vi "Combination_Digitizer_Driver - REWORK.vi"(0 "Mode":T5(ring), 1 "Horizontal Settings":T2={"number of records"=1, "reference position"=50.0, "min record length"=50000, "min sample rate"=200000.0, "enforce realtime"=FALSE, "maximum input frequency"=0.0} {"maximum input frequency" format="%.2f"; "min sample rate" step=1000000.0; "reference position" format="%.1f"; "number of records" step=1}, 2 "Vertical Settings":T4={"vertical coupling"=enum."DC", "probe attenuation"=20.0, "vertical range"=120.0, "vertical offset"=0.0} {"vertical offset" format="%.4f"; "vertical range" format="%.2f"; "probe attenuation" format="%.1f"}, 3 "Trigger Settings":T3={"trigger level"=30.0, "trigger type"=enum."Edge", "Trigger Source"=enum."Channel 0", "Trigger Slope"=enum."Positive"} {"trigger level" format="%.2f"}, 5 "Channel Name":string="0", 11 "error in":errorcluster) -> (6 "Waveform Array":waveform(dbl)[](array[waveform]), 8 "Ch1_Plot":dbl[](array[numeric]), 15 "error out":errorcluster)   [LabVIEW 2010]
uses:
  Typedef-Channel Parameters.ctl
panel:
  in  "Channel Parameters In":T1={"Channel Name"="0", "Number of Records"=0, "Reference Position"=0.0, "Minimum Record Length"=0, "Minimum Sample Rate"=0.0, "Maximum Input Frequency"=0.0, "Enforce Realtime"=FALSE, "Vertical Coupling"=enum."AC", "Probe Attenuation"=0.0, "Vertical Range (V)"=0.0, "Vertical Offset"=0.0, "Trigger Level"=0.0, "Trigger Type"=enum."Edge", "Trigger Source"=enum."Immediate", "Trigger Slope"=enum."Positive", "Digitizer 1 Used?"=FALSE, "Digitizer 1 Channels"="", "Digitizer 1 Reference"="", "Digitizer 1 Gain Multiplier"=nan, "Digitizer 2 Used?"=FALSE, "Digitizer 2 Channels"="", "Digitizer 2 Reference"="", "Session References"=[]}
  out "Channel Parameters":T1={"Channel Name"="0", "Number of Records"=0, "Reference Position"=0.0, "Minimum Record Length"=0, "Minimum Sample Rate"=0.0, "Maximum Input Frequency"=0.0, "Enforce Realtime"=FALSE, "Vertical Coupling"=enum."AC", "Probe Attenuation"=0.0, "Vertical Range (V)"=0.0, "Vertical Offset"=0.0, "Trigger Level"=0.0, "Trigger Type"=enum."Edge", "Trigger Source"=enum."Immediate", "Trigger Slope"=enum."Positive", "Digitizer 1 Used?"=FALSE, "Digitizer 1 Channels"="", "Digitizer 1 Reference"="", "Digitizer 1 Gain Multiplier"=nan, "Digitizer 2 Used?"=FALSE, "Digitizer 2 Channels"="", "Digitizer 2 Reference"="", "Session References"=[]}
  out "Waveform":T6(graph)
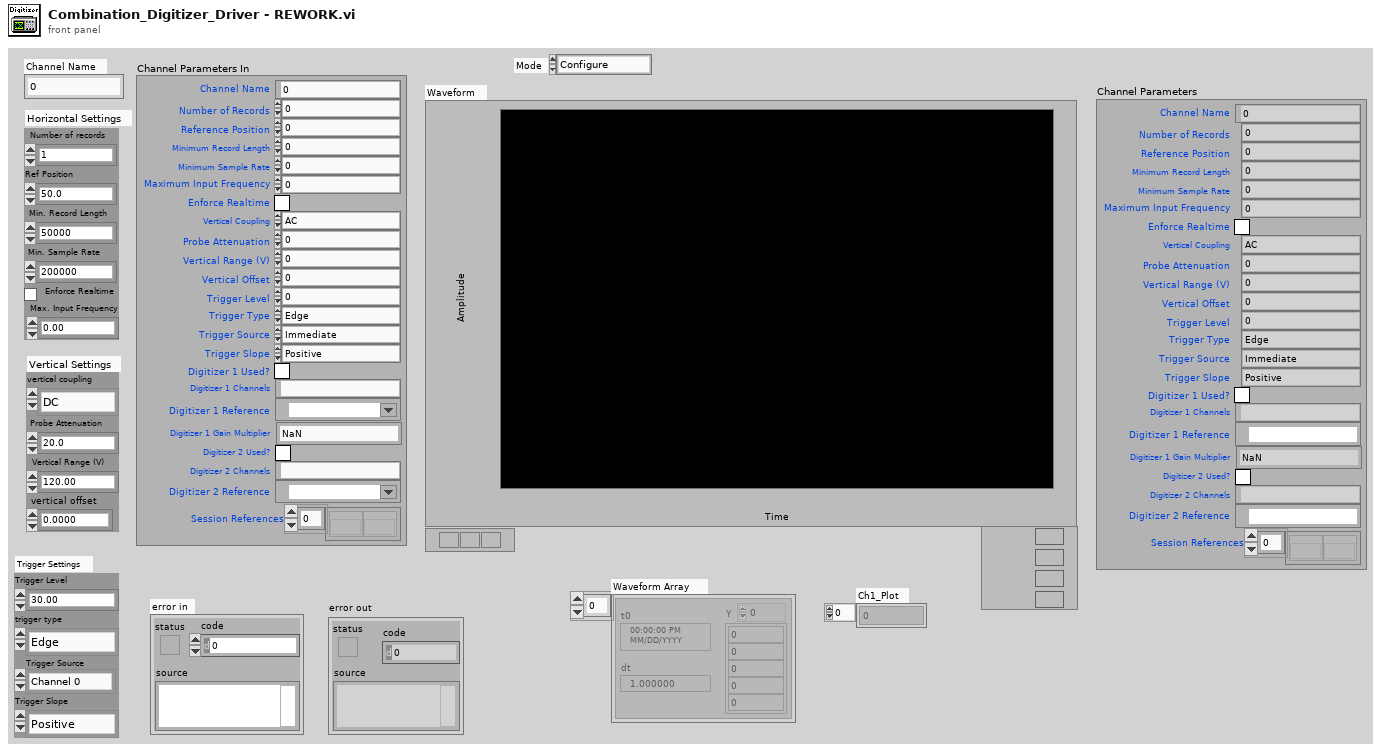
[diagram p1: front panel]
types:
  T1 = typedef "Typedef-Channel Parameters.ctl" = cluster{"Channel Name":string, "Number of Records":i32, "Reference Position":dbl, "Minimum Record Length":i32, "Minimum Sample Rate":dbl, "Maximum Input Frequency":dbl, "Enforce Realtime":bool, "Vertical Coupling":enum16{"AC", "DC", "Ground"}, "Probe Attenuation":dbl, "Vertical Range (V)":dbl, "Vertical Offset":dbl, "Trigger Level":dbl, "Trigger Type":enum16{"Edge", "Digital", "Immediate"}, "Trigger Source":enum16{"Immediate", "Channel 0", "Channel 1", "Channel 2", "Channel 3", "Channel 4", "Channel 5", "Channel 6", "Channel 7", "Extermal TRIG", "Software Trigger", "RTSI 0", "RTSI 1", "RTSI 2", "RTSI 3", "RTSI 4", "RTSI 5", "RTSI 6", "PF 0", "PF 1", "PF 2", "PXI Star Trigger"}, "Trigger Slope":enum16{"Positive", "Negative"}, "Digitizer 1 Used?":bool, "Digitizer 1 Channels":string, "Digitizer 1 Reference":refnum<k15>, "Digitizer 1 Gain Multiplier":dbl, "Digitizer 2 Used?":bool, "Digitizer 2 Channels":string, "Digitizer 2 Reference":refnum<k15>, "Session References":refnum<k20>[]}
  T2 = cluster{"number of records":i32, "reference position":dbl, "min record length":i32, "min sample rate":dbl, "enforce realtime":bool, "maximum input frequency":dbl}
  T3 = cluster{"trigger level":dbl, "trigger type":enum16{"Edge", "Digital", "Immediate"}, "Trigger Source":enum8{"Immediate", "Channel 0", "Channel 1", "Channel 2", "Channel 3", "Channel 4", "Channel 5", "Channel 6", "Channel 7", "External TRIG", "Software Trigger", "RTSI 0", "RTSI 1", "RTSI 2", "RTSI 3", "RTSI 4", "RTSI 5", "RTSI 6", "PFI 0", "PFI 1", "PFI 2", "PXI Star Trigger"}, "Trigger Slope":enum16{"Positive", "Negative"}}
  T4 = cluster{"vertical coupling":enum16{"AC", "DC", "Ground"}, "probe attenuation":dbl, "vertical range":dbl, "vertical offset":dbl}
  T5 = enum16{"Configure", "Read", "TriggerRead", "Close", "Init"}
  T6 = cluster{"relativeInitialX":dbl, "xIncrement":dbl, "wfm":dbl[]}[]
  T7 = cluster{"Channel Name":string, "Number of Records":i32, "Reference Position":dbl, "Minimum Record Length":i32, "Minimum Sample Rate":dbl, "Maximum Input Frequency":dbl, "Enforce Realtime":bool, "Vertical Coupling":enum16{"AC", "DC", "Ground"}, "Probe Attenuation":dbl, "Vertical Range (V)":dbl, "Vertical Offset":dbl, "Trigger Level":dbl, "Trigger Type":enum16{"Edge", "Digital", "Immediate"}, "Trigger Source":enum16{"Immediate", "Channel 0", "Channel 1", "Channel 2", "Channel 3", "Channel 4", "Channel 5", "Channel 6", "Channel 7", "Extermal TRIG", "Software Trigger", "RTSI 0", "RTSI 1", "RTSI 2", "RTSI 3", "RTSI 4", "RTSI 5", "RTSI 6", "PF 0", "PF 1", "PF 2", "PXI Star Trigger"}, "Trigger Slope":enum16{"Positive", "Negative"}, "Digitizer 1 Used?":bool, "Digitizer 1 Channels":string, "Digitizer 1 Reference":refnum<k15>, "Digitizer 1 Gain Multiplier":dbl, "Digitizer 2 Used?":bool, "Digitizer 2 Channels":string, "Digitizer 2 Reference":refnum<k15>, "Session References":refnum<k20>[]}
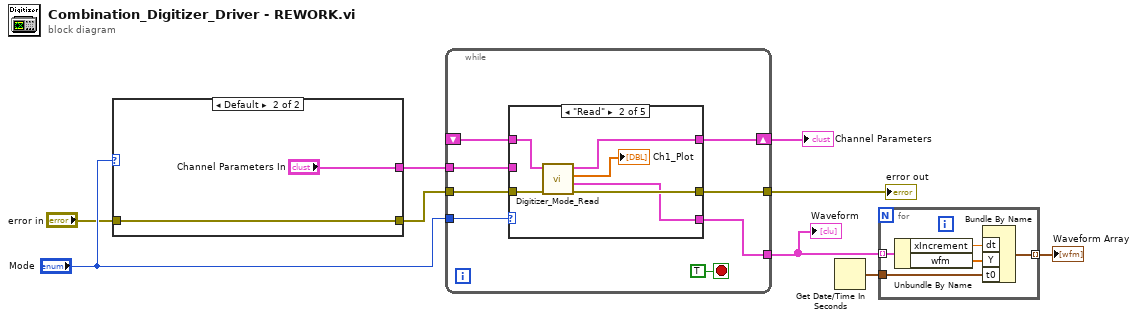
[diagram p0: block diagram]
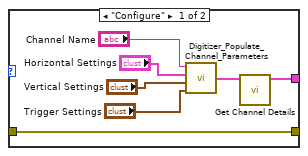
[diagram p2: hidden frame]
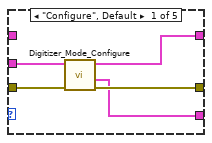
[diagram p3: hidden frame]
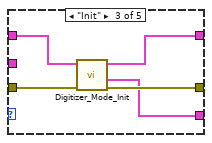
[diagram p4: hidden frame]
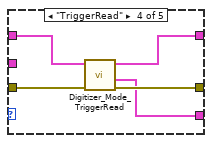
[diagram p5: hidden frame]
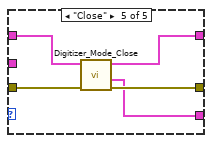
[diagram p6: hidden frame]
diagram:
  n1 = case shown="Default" "Mode" {
    tunnel: [w11 "Channel Parameters In"] -> w5
    tunnel: "error in" -> [w10 w18]
    tunnel: [w10 w18] -> w1
    frame "Configure" {
      n2 = call "Digitizer_Populate_Channel_Parameters"("Trigger settings"="Trigger Settings", "Vertical Settings"="Vertical Settings", "Horizontal Settings"="Horizontal Settings", "Channel Name"="Channel Name") -> ("Channel Parameters"=w12:T1)
      n3 = call "Get Channel Details.vi"("Channel Parameters In"=w12) -> ("Channel Parameters Out"=w11:T1)  [unwired: 10 in]
    }
    frame Default {
    }
  }
  n4 = while {
    tunnel: "Mode" -> [w25]
    shift-right: [w23] -> w4
    shift-left: _ -> [w24]
    tunnel: w1 -> [w22]
    tunnel: [w21] -> w9
    tunnel: [w20] -> w8
    tunnel: w5 -> [w19]
    stop <- TRUE stop-if-true
    n5 = case shown="\"Read\"" w25 {
      tunnel: w24 -> [_ w32 w38 w43 w49]
      tunnel: [w27 w33 w40 w45 w48] -> w23
      tunnel: w22 -> [w30 w37 w42 w47 w51]
      tunnel: [w29 w36 w41 w46 w52] -> w21
      tunnel: [w28 w35 w39 w44 w50] -> w20
      tunnel: w19 -> [w31 _ _ _ _]
      frame "Configure", Default {
        n6 = call "Digitizer_Mode_Configure.vi"("error in"=w30, "Channel Parameters In"=w31) -> ("error out"=w29:errorcluster, "Waveforms Out (Empty)"=w28:T6, "Channel Parameters Out"=w27:T1)  [unwired: 7 in]
      }
      frame "Read" {
        n7 = call "Digitizer_Mode_Read.vi"("error in"=w37, "Channel Parameters In"=w32) -> ("error out"=w36:errorcluster, "Waveforms Out"=w35:T6, "Ch1_Plot"=→"Ch1_Plot":dbl[], "dup Channel Parameters Out"=w33:T1)  [unwired: 6 in]
      }
      frame "Init" {
        n8 = call "Digitizer_Mode_Init.vi"("error in"=w42, "Channel Parameters In"=w38) -> ("error out"=w41:errorcluster, "Waveforms Out (Empty)"=w39:T6, "dup Channel Parameters Out"=w40:T1)  [unwired: 7 in]
      }
      frame "TriggerRead" {
        n9 = call "Digitizer_Mode_TriggerRead.vi"("error in"=w47, "Channel Parameters In"=w43) -> ("error out"=w46:errorcluster, "Waveforms Out"=w44:T6, "dup Channel Parameters Out"=w45:T1)  [unwired: 7 in]
      }
      frame "Close" {
        n10 = call "Digitizer_Mode_Close.vi"("error in"=w51, "Channel Parameters In"=w49) -> ("error out"=w52:errorcluster, "Waveforms Out (Empty)"=w50:T6, "Channel Parameters Reset"=w48:T7)  [unwired: 7 in]
      }
    }
  }
  "error out" <- w9
  "Waveform" <- w8
  "Channel Parameters" <- w4
  n11 = Get Date/Time In Seconds() -> (seconds since 1Jan1904=w6:timestamp)
  n12 = for {
    tunnel: w8 -> [w57] mode=indexing
    tunnel: [w54] -> w7 mode=indexing
    tunnel: w6 -> [w53]
    n13 = Unbundle By Name(w57) -> ("xIncrement"=w56:dbl, "wfm"=w55:dbl[])
    n14 = Bundle By Name("dt"=w56, "Y"=w55, "t0"=w53) -> (w54:waveform(dbl))  [unwired: 1 in]
  }
  "Waveform Array" <- w7
